vi "Test_Ethernet_Camera_F1.vi"() -> ()   [LabVIEW 2024]
uses:
  <vilib>/vision/driver/NI_Vision_Acquisition_Software.lvlib
  <vilib>/vision/NI_Vision_Development_Module.lvlib
panel:
  out "Image":T1(plugin-control)
  out "error out 2":errorcluster
  in  "Take calibration picture":bool
  out "Camera Information Array":T2(array[cluster]) {"BusType" format="%x"; "SerialNumberLow" format="%.0x"; "SerialNumberHigh" format="%.0x"}
  out "error out":errorcluster
  out "InterfaceName":string
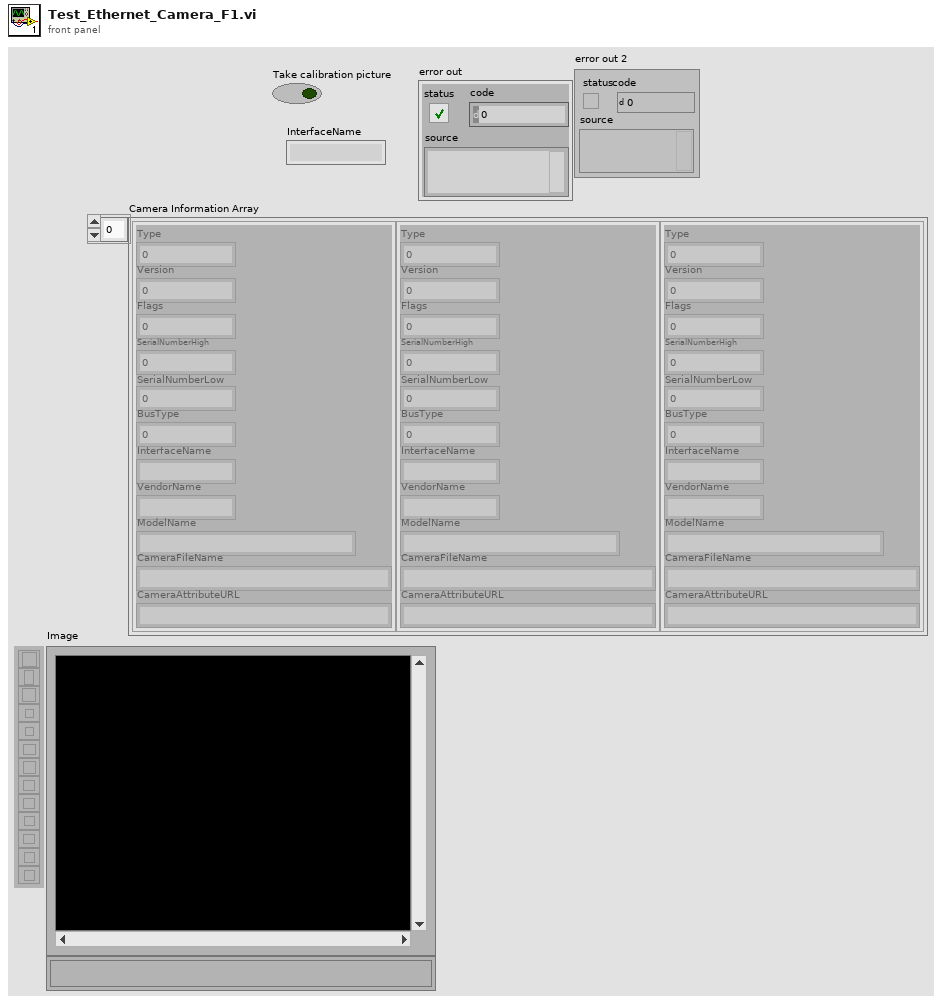
[diagram p1: front panel]
types:
  T1 = typedef "IMAQ Image.ctl" = refnum<image>
  T2 = cluster{"Type":u32, "Version":u32, "Flags":u32, "SerialNumberHigh":u32, "SerialNumberLow":u32, "BusType":u32, "InterfaceName":string, "VendorName":string, "ModelName":string, "CameraFileName":string, "CameraAttributeURL":string}[]
  T3 = typedef "Image Type" = u32
  T4 = typedef "IMAQdx.ctl" = refnum<k21>
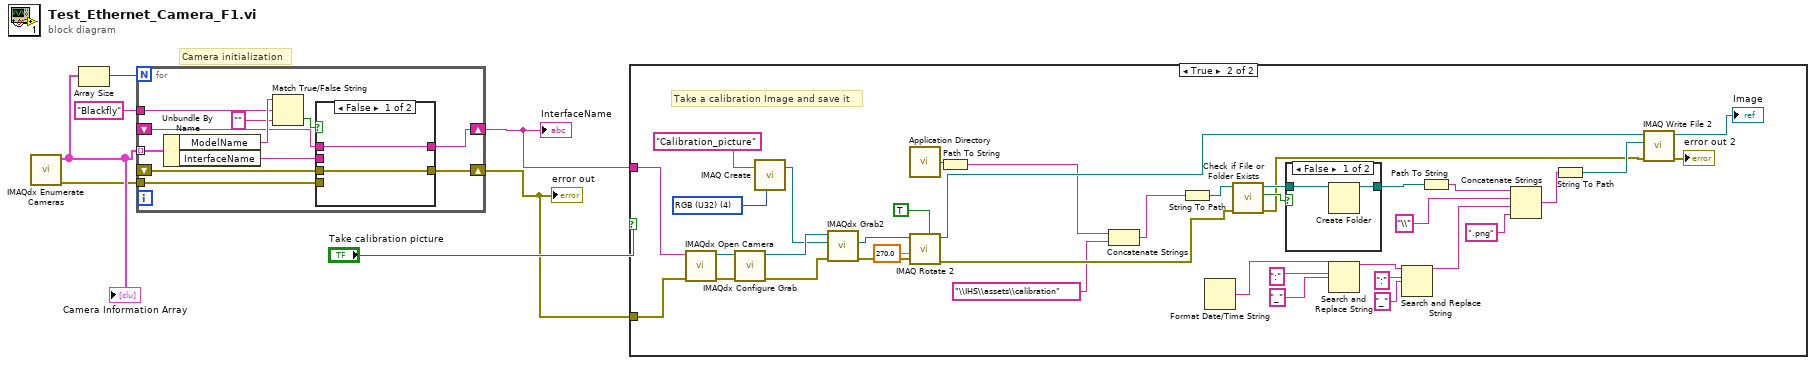
[diagram p0: block diagram]
diagram:
  # "Camera initialization"
  n1 = call <vilib>:"IMAQdx Enumerate Cameras.vi"() -> ("error out"=w5:errorcluster, "Camera Information Array"=w6:T2)  [unwired: 10 in]
  "Camera Information Array" <- w6
  n2 = Array Size(array=w6) -> (size(s)=w7:i32)
  n3 = for {
    N: w7 -> [_]
    tunnel: w6 -> [w18] mode=indexing
    tunnel: w5 -> [w13]
    tunnel: "Blackfly" ("regular expression") -> [w15]
    shift-right: [w10] -> w1
    shift-left: _ -> [w9]
    shift-right: [w12] -> w2
    shift-left: _ -> [w11]
    n4 = Unbundle By Name(w18) -> ("ModelName"=w16:string, "InterfaceName"=w17:string)
    n5 = Match True/False String(2:"" ("false string"), 3:w15, 4:w16) -> (0:w14:bool)  [unwired: 1 out]
    n6 = case shown="False" w14 {
      tunnel: w17 -> [_ w22]
      tunnel: [w20 w22] -> w12
      tunnel: w13 -> [_ w21]
      tunnel: [w19 w21] -> w10
      tunnel: w11 -> [w20 _]
      tunnel: w9 -> [w19 _]
      frame False {
      }
      frame True {
      }
    }
  }
  "InterfaceName" <- w2
  "error out" <- w1
  n7 = case shown="True" "Take calibration picture" {
    tunnel: w2 -> [_ w56]
    tunnel: w1 -> [_ w55]
    frame False {
    }
    frame True {
      w57 = T3 4 items=["Grayscale (U8)", "Grayscale (I16)", "Grayscale (SGL)", "Complex (CSG)", "RGB (U32)", "HSL (U32)", "RGB (U64)", "Grayscale (U16)"] ("Image Type")
      # "Take a calibration Image and save it"
      n8 = call <vilib>:"IMAQdx Open Camera.vi"("error in"=w55, "Session In"=w56) -> ("error out"=w59:errorcluster, "Session Out"=w60:T4)  [unwired: 8 in]
      n9 = call <vilib>:"IMAQdx Configure Grab.vi"("error in"=w59, "Session In"=w60) -> ("error out"=w52:errorcluster, "Session Out"=w54:T4)  [unwired: 8 in]
      n10 = call "IMAQ Create"("Image Name"="Calibration_picture", "Image Type"=w57) -> ("New Image"=w53:T1)  [unwired: 3 in, 1 out]
      n11 = call <vilib>:"IMAQdx Grab2.vi"("error in"=w52, "Image In"=w53, "Session In"=w54) -> ("error out"=w51:errorcluster, "Image Out"=w24:T1)  [unwired: 5 in, 2 out]
      n12 = call <vilib>:"Application Directory.vi"() -> ("Application Directory"=w48:path)
      n13 = call "IMAQ Rotate 2"("Maintain Size"=TRUE, "error in (no error)"=w51, "Angle (degrees)"=270.0, "Image Src"=w24) -> ("error out"=w30:errorcluster, "Image Dst Out"=w33:T1)  [unwired: 6 in]
      n14 = Path To String(path=w48) -> (string=w29:string)
      n15 = Concatenate Strings(w29, "\\IHS\\assets\\calibration" ("string")) -> (w47:string)
      n16 = String To Path(string=w47) -> (path=w27:path)
      n17 = Format Date/Time String() -> (date/time string=w23:string)  [unwired: 3 in]
      n18 = call <vilib>:"Check if File or Folder Exists.vi"("error in (no error)"=w30, "path"=w27) -> ("error out"=w31:errorcluster, "file or folder exists?"=w44:bool, "dup path"=w43:path)  [unwired: 7 in]
      n19 = case shown="False" w44 {
        tunnel: w43 -> [w62 w63]
        tunnel: [w61 w63] -> w45
        frame False {
          n20 = Create Folder(path (use dialog)=w62) -> (created path=w61:path)  [unwired: 2 in, 2 out]
        }
        frame True {
        }
      }
      n21 = Search and Replace String(input string=w23, search string=":", replace string="_" ("replace string (\"\")")) -> (result string=w35:string)  [unwired: 5 in, 3 out]
      n22 = Search and Replace String(input string=w35, search string=":", replace string="_" ("replace string (\"\")")) -> (result string=w34:string)  [unwired: 5 in, 3 out]
      n23 = Path To String(path=w45) -> (string=w41:string)
      n24 = Concatenate Strings(w41, "\\" ("string"), w34, ".png" ("string")) -> (w46:string)
      n25 = String To Path(string=w46) -> (path=w32:path)
      n26 = call-poly "IMAQ Write File 2"("error in (no error)"=w31, "File Path"=w32, "Image"=w33) -> ("error out"=→"error out 2":errorcluster, "Image Out (duplicate)"=→"Image":T1)  [unwired: 7 in]
    }
  }
